vi "输入读取.vi"() -> (3 "输入":T1)   [LabVIEW 2017]
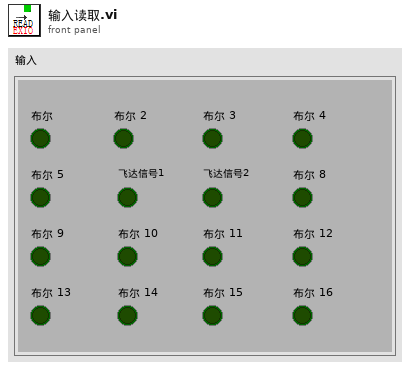
[diagram p1: front panel]
types:
  T1 = typedef "input控件.ctl" = cluster{"布尔":bool, "布尔 2":bool, "布尔 3":bool, "布尔 4":bool, "布尔 5":bool, "飞达信号1":bool, "飞达信号2":bool, "布尔 8":bool, "布尔 9":bool, "布尔 10":bool, "布尔 11":bool, "布尔 12":bool, "布尔 13":bool, "布尔 14":bool, "布尔 15":bool, "布尔 16":bool}
  T2 = typedef "配置检索操作.ctl" = enum16{"配置检索", "名称提取", "寄存器提取"}
  T3 = typedef "输入&输出配置提取集合.ctl" = cluster{"IO配置名称":string[], "IO配置点位地址":string[], "IO配置名称索引":i32[], "取反信息":i32[], "簇属性集合":string[]}
  T4 = cluster{"[0]":bool, "[1]":bool, "[2]":bool, "[3]":bool, "[4]":bool, "[5]":bool, "[6]":bool, "[7]":bool, "[8]":bool, "[9]":bool, "[10]":bool, "[11]":bool, "[12]":bool, "[13]":bool, "[14]":bool, "[15]":bool}
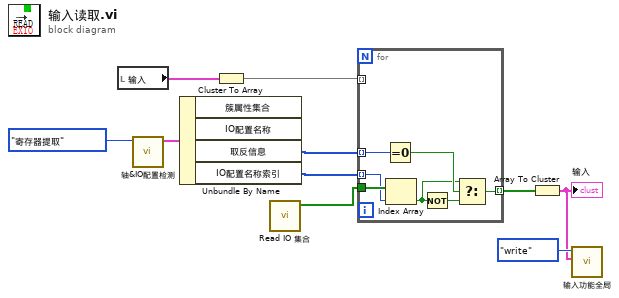
[diagram p0: block diagram]
diagram:
  n1 = local read "输入"() -> (w4:T1)
  n2 = call "轴&IO配置检测.vi"("配置检索操作"=配置检索操作."寄存器提取") -> ("输入配置提取集合"=w5:T3)  [unwired: 8 in, 2 out]
  n3 = Unbundle By Name(w5) -> ("取反信息"=w7:i32[], "IO配置名称索引"=w8:i32[])  [unwired: 2 out]
  n4 = Cluster To Array(cluster=w4) -> (array=w3:bool[])
  n5 = call "Read IO 集合.vi"() -> ("IO集合"=w10:bool[])  [unwired: 11 in]
  n6 = for {
    tunnel: w8 -> [w16] mode=indexing
    tunnel: w10 -> [w17]
    tunnel: w7 -> [w15] mode=indexing
    tunnel: w3 -> [_] mode=indexing
    tunnel: [w11] -> w1 mode=indexing
    n7 = Equal To 0?(x=w15) -> (x = 0?=w14:bool)
    n8 = Index Array(array=w17, index=w16) -> (element=w13:bool)
    n9 = Not(x=w13) -> (.not. x?=w12:bool)
    n10 = Select(t=w13, s=w14, f=w12) -> (s? t:f=w11:bool)
  }
  n11 = Array To Cluster(array=w1) -> (cluster=w2:T4)
  "输入" <- w2
  n12 = call "输入功能全局.vi"("输入"=w2, "选项"=enum16{"initialize", "read", "write"}."write") -> ()  [unwired: 9 in, 1 out]
